vi "Get HTTP Method.vi"(8 "Error In":errorcluster, 9 "Enum":T1) -> (0 "error out":errorcluster, 1 "HTTPMethod":refnum<k24>)   [LabVIEW 2018, in "LabVIEWHTTPClient_NET.lvlib" / "HttpRequestMessage.lvclass"]
uses:
  HttpRequestMessage.lvclass
  System.Net.Http
  Types/method_enum.ctl
  LabVIEWHTTPClient_NET/LabVIEWHTTPClient_NET.lvlib
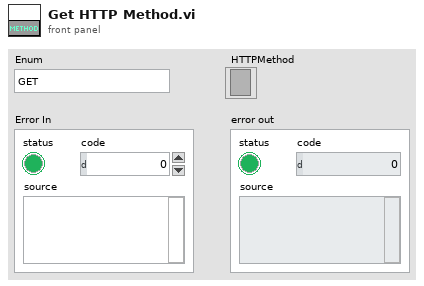
[diagram p1: front panel]
types:
  T1 = typedef "LabVIEWHTTPClient_NET.lvlib/method_enum.ctl" = enum16{"GET", "PUT", "POST", "DELETE", "HEAD", "TRACE", "SEND"}
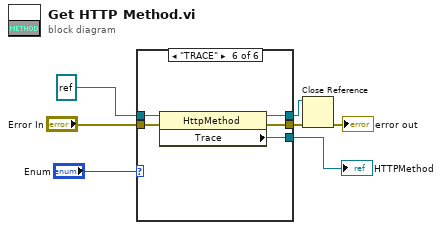
[diagram p0: block diagram]
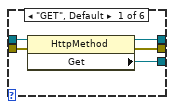
[diagram p2: hidden frame]
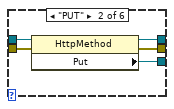
[diagram p3: hidden frame]
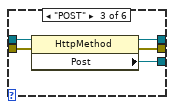
[diagram p4: hidden frame]
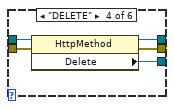
[diagram p5: hidden frame]
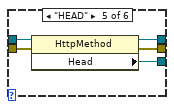
[diagram p6: hidden frame]
diagram:
  n1 = case shown="\"TRACE\"" "Enum" {
    tunnel: refnum<k24> refnum ("reference") -> [w12 w17 w22 w27 w32 w37]
    tunnel: [w9 w16 w21 w26 w31 w36] -> w6
    tunnel: [w11 w15 w20 w25 w30 w35] -> w3
    tunnel: [w10 w14 w19 w24 w29 w34] -> w4
    tunnel: "Error In" -> [w8 w13 w18 w23 w28 w33]
    frame "GET", Default {
      n2 = property class="HttpMethod"(reference=w12, error in=w8) -> (reference out=w11:refnum<k24>, error out=w10:errorcluster, "Get"=w9:refnum<k24>)
    }
    frame "PUT" {
      n3 = property class="HttpMethod"(reference=w17, error in=w13) -> (reference out=w15:refnum<k24>, error out=w14:errorcluster, "Put"=w16:refnum<k24>)
    }
    frame "POST" {
      n4 = property class="HttpMethod"(reference=w22, error in=w18) -> (reference out=w20:refnum<k24>, error out=w19:errorcluster, "Post"=w21:refnum<k24>)
    }
    frame "DELETE" {
      n5 = property class="HttpMethod"(reference=w27, error in=w23) -> (reference out=w25:refnum<k24>, error out=w24:errorcluster, "Delete"=w26:refnum<k24>)
    }
    frame "HEAD" {
      n6 = property class="HttpMethod"(reference=w32, error in=w28) -> (reference out=w30:refnum<k24>, error out=w29:errorcluster, "Head"=w31:refnum<k24>)
    }
    frame "TRACE" {
      n7 = property class="HttpMethod"(reference=w37, error in=w33) -> (reference out=w35:refnum<k24>, error out=w34:errorcluster, "Trace"=w36:refnum<k24>)
    }
  }
  "HTTPMethod" <- w6
  n8 = Close Reference(reference=w3, error in (no error)=w4) -> (error out=→"error out":errorcluster)
